vi "commander9.vi"() -> ()   [LabVIEW 2015]
uses:
  <vilib>/National Instruments/NI Dynamixel API/Dynamixel Pro Driver/Controls/Write Select Pro.ctl
  <vilib>/National Instruments/NI Dynamixel API/Dynamixel Pro Driver/Controls/Baudrate Selector.ctl
  G_ALL.vi
  G_LCM.vi
  G_SEN.vi
  <vilib>/National Instruments/NI Dynamixel API/Dynamixel Pro Driver/Write/Write Dynamixel Pro.vi
  <vilib>/National Instruments/NI Dynamixel API/Dynamixel Pro Driver/Helper VIs/Torque Disable.vi
  <vilib>/National Instruments/NI Dynamixel API/Dynamixel Pro Driver/Helper VIs/Torque Enable.vi
  <vilib>/National Instruments/NI Dynamixel API/Dynamixel Pro Driver/Dynamixel Pro Driver.lvlib
panel:
  in  "Mission":i32
  out "size(s)":i32
  in  "shiift torque gain":i32
  out "robotis":refnum<visa-resource-name>
  in  "y 2":dbl=1.0
  in  "y":dbl=0.5 format="%#_13g"
  out "CIPV_dist":dbl
  out "CIPV_SPEED":dbl
  in  "dist_error_gain":dbl=0.5 format="%#_13g"
  in  "Globla y shift":dbl min=-5.0 max=5.0 step=0.1
  in  "d":dbl=-3.5 format="%#_13g"
  in  "car detection":bool
  in  "Velodyne":T1(ring)=enum."Velodyne 64"
  in  "reset path":bool
  in  "shifthold":dbl=0.003
  out "String":string
  out "EURECAR_VISION":T2
  out "count":i32=100
  out "P2V Sign":picture[](array[picture])=[bytes[7530], bytes[7530], bytes[7530], bytes[7530]]
  out "Array 2":picture[](array[picture])
  out "sign 2":picture[](array[picture])=[bytes[7530], bytes[7530], bytes[7530], bytes[7530], bytes[7530], bytes[7530]]
  out "sign":picture[](array[picture])=[bytes[14730], bytes[14730], bytes[14730], bytes[14730], bytes[14730], bytes[14730], bytes[14730]]
  in  "TTL":bool=TRUE
  out "obs shift":dbl format="%.2f"
  in  "lane keep":bool=TRUE
  in  "replay":bool
  in  "Global x shift":dbl min=-5.0 max=5.0 step=1.0
  out "display":u32=33
  out "control":u32=10
  out "lane update":bool=TRUE
  in  "save lcm":bool
  out "LCM Recv Data":string="LCM_SELF_TEST\t2\rIBEO_2202_T\t29020\rSDT_GPS_DATA\t5359\rGGA_1\t5359\rRMC_1\t5359\rMobileye560\t14820\rPOS_T\t116849\rPATH_T\t116934\rCON_T\t116934\rVELO_384\t1693774\rCAN_T\t116936\rSantafe\t116936\r"
  out "GPS DATA 2":T3={"type"="WAAS", "x_lcc"=254.06227375244842, "y_lcc"=-1012.895186102979, "latdev"=0.63, "londev"=0.63, "sats"=12, "gps_l1_ranges"=0, "gps_l1_mask_ranges"=0, "gps_l2_mask_ranges"=0, "Heading"=246.4954324105635, "lon"=127.36372, "lat"=36.36631, "time"="22:33:04.0", "hgps"=245.36, "lag"=0.0, "MAP"="KAIST"} {"lag" format="%#_5g"; "hgps" format="%#_5g"; "lat" format="%#_11g"; "lon" format="%#_11g"; "Heading" format="%#_5g"; "latdev" format="%#_4g"; "londev" format="%#_4g"}
  in  "Obs":bool=TRUE
  in  "Log":bool=TRUE
  out "path":u32=10
  out "sensor":u32=10 format="%02.0f"
  out "Speed limit":dbl=25.0
  out "collision":bool
  in  "Load Path":bool
  in  "Max. Vel.":dbl=10.0 min=-5.0 max=120.0 step=5.0
  out "col":i16(graph)
  out "stop":bool=TRUE
  in  "Reverse":bool
  in  "STOP":bool
  out "Waveform Chart 4":cluster{"auto":i16, "run":i16}(graph)={"auto"=1, "run"=0}
  out "Waveform Chart 3":cluster{"Steer_input":dbl, dbl, "handle":dbl}(graph)={"Steer_input"=-0.0, 31.6, "handle"=6.530305819273729}
  out "Waveform Chart 2":T4(graph)={"VS_des"=0.0, "VS_can"=22.140625, "VS_des"=0.0}
  out "Heading":cluster{"Heading":dbl, "hgps":dbl}(graph)={"Heading"=246.4954324105635, "hgps"=245.36}
  out "XY Graph 2":cluster{"Y":dbl[], "Y":dbl[]}[](graph)=[{"Y"=[254.2844178548139], "Y"=[-1012.8240977739181]}, {"Y"=array[3210 elements], "Y"=array[3210 elements]}, {"Y"=array[3210 elements], "Y"=array[3210 elements]}]
  out "Gauge":cluster{dbl, dbl, dbl}(knob)={0.0, 22.140625, 0.0} scale=-20.0..140.0
  out "Meter":cluster{dbl, dbl, dbl}(knob)={-0.0, 31.6, 6.530305819273729} scale=-550.0..550.0
  out "XY Graph":cluster{"Y":dbl[], "Y":dbl[]}[](graph)=[{"Y"=array[3210 elements], "Y"=array[3210 elements]}, {"Y"=[-0.0, 0.001154394197769193, 0.004617650635850623, 0.010389990872226917, 0.018471784248973222, 0.02886354801042046, 0.041565947468740205, 0.056579796217107514, 0.0739060563904701, 0.0935458389742223, 0.11550040416098284, 0.13977116175580306, 0.16635967162997645, 0.19526764422393228, 0.2264969410994837, 0.26004957554195585, 0.2959277132125635, 0.3341336728515216, 0.374669927032528, 0.417539102969144, 0.4627439833735707, 0.5102875073687159, 0.560172771454063, 0.6124030305261954, 0.6669816989546717, 0.7239123517142048, 0.7831987255740245, 0.8448447203451934, 0.9088544001870815, 0.975231994973953, 1.0439819017227023, 1.1151086860829622, 1.1886170838907617, 1.2645120027869723, 1.342798523901962, 1.42348190360768, 1.5065675753387922, 1.592061151484188, 1.6799684253507792, 1.770295373200753, 1.8630481563645134, 1.9582331234307588, 2.0558568125157564, 2.1559259536137603, 2.258447471030621], "Y"=[0.0, 0.5, 1.0, 1.5, 2.0, 2.5, 3.0, 3.5, 4.0, 4.5, 5.0, 5.5, 6.0, 6.5, 7.0, 7.5, 8.0, 8.5, 9.0, 9.5, 10.0, 10.5, 11.0, 11.5, 12.0, 12.5, 13.0, 13.5, 14.0, 14.5, 15.0, 15.5, 16.0, 16.5, 17.0, 17.5, 18.0, 18.5, 19.0, 19.5, 20.0, 20.5, 21.0, 21.5, 22.0]}, {"Y"=[0.362252581831572], "Y"=[-0.8199241909738847]}, {"Y"=array[210 elements], "Y"=array[210 elements]}, {"Y"=[-0.925, -0.925, -0.925, -0.6775, -0.6775, -0.925, -0.925, -0.925, -0.925, -0.6775, -0.6775, -0.925, -0.925, -0.925, 0.9025, 0.9025, 0.9025, 0.6775, 0.6775, 0.9025, 0.9025, 0.9025, 0.9025, 0.6775, 0.6775, 0.9025, 0.9025, 0.9025, -0.925], "Y"=[-0.75, -0.224, 0.224, 0.224, -0.224, -0.224, 0.224, 2.415, 2.885, 2.885, 2.415, 2.415, 2.885, 3.5, 3.5, 2.885, 2.415, 2.415, 2.885, 2.885, 2.415, 0.224, -0.224, -0.224, 0.224, 0.224, -0.224, -0.75, -0.75]}, {"Y"=[0.171875, 0.15377271904051304, 0.1346290179491043, 0.11445423440635205, 0.09325870609283447, 0.07105277068912982, 0.04784676587581635, 0.02365102933347224, -0.0015241012573242174, -0.02766828821599482, -0.05477119386196136, -0.08282248051464558, -0.11181181049346922, -0.14172884611785413, -0.17256324970722198, -0.20430468358099463, -0.23694281005859374, -0.27046729145944115, -0.30486779010295867, -0.340133968308568, -0.3762554883956909, -0.41322201268374914, -0.4510232034921646, -0.4896487231403589], "Y"=[0.0, 0.5, 1.0, 1.5, 2.0, 2.5, 3.0, 3.5, 4.0, 4.5, 5.0, 5.5, 6.0, 6.5, 7.0, 7.5, 8.0, 8.5, 9.0, 9.5, 10.0, 10.5, 11.0, 11.5]}, {"Y"=[1.796875, 1.778772719040513, 1.7596290179491043, 1.739454234406352, 1.7182587060928345, 1.6960527706891297, 1.6728467658758164, 1.6486510293334722, 1.6234758987426758, 1.5973317117840051, 1.5702288061380387, 1.5421775194853544, 1.513188189506531, 1.483271153882146, 1.452436750292778, 1.4206953164190055, 1.3880571899414063, 1.354532708540559, 1.3201322098970414, 1.284866031691432, 1.248744511604309, 1.2117779873162509, 1.1739767965078354, 1.135351276859641, 1.0959117660522462, 1.0556686017662287, 1.014632121682167, 0.9728126634806396, 0.9302205648422242, 0.8868661634474992], "Y"=[0.0, 0.5, 1.0, 1.5, 2.0, 2.5, 3.0, 3.5, 4.0, 4.5, 5.0, 5.5, 6.0, 6.5, 7.0, 7.5, 8.0, 8.5, 9.0, 9.5, 10.0, 10.5, 11.0, 11.5, 12.0, 12.5, 13.0, 13.5, 14.0, 14.5]}, {"Y"=[-1.453125, -1.471227280959487, -1.4903709820508957, -1.510545765593648, -1.5317412939071655, -1.5539472293108703, -1.5771532341241836, -1.6013489706665278, -1.6265241012573242, -1.6526682882159949, -1.6797711938619613, -1.7078224805146456, -1.736811810493469, -1.766728846117854, -1.797563249707222, -1.8293046835809945, -1.8619428100585937, -1.895467291459441, -1.9298677901029586], "Y"=[0.0, 0.5, 1.0, 1.5, 2.0, 2.5, 3.0, 3.5, 4.0, 4.5, 5.0, 5.5, 6.0, 6.5, 7.0, 7.5, 8.0, 8.5, 9.0]}, {"Y"=[0.171875, 0.2568230007600336, 0.3384052130063493, 0.44574342526006827, 0.5205081969556753, 0.5917680690742042, 0.659409530134929, 0.7229937549325056, 0.7835496148685115, 0.8405449546633443, 0.9258576868463875], "Y"=[-20.239964538708662, -19.725637940364884, -19.211158961966362, -18.6998967366845, -18.19022720070031, -17.681887266143153, -17.17615515566314, -16.67683575591291, -16.176265245349786, -15.679082775270938, -15.183754484614711]}, {"Y"=[7.134647485270904], "Y"=[38.71960961082238]}, {"Y"=array[980 elements], "Y"=array[980 elements]}, {"Y"=[], "Y"=[]}]
  in  "Make WPT":bool
  in  "mission auto":bool
  # "V2I Traffic Signal"
  # "CNN\nSign\nDetection"
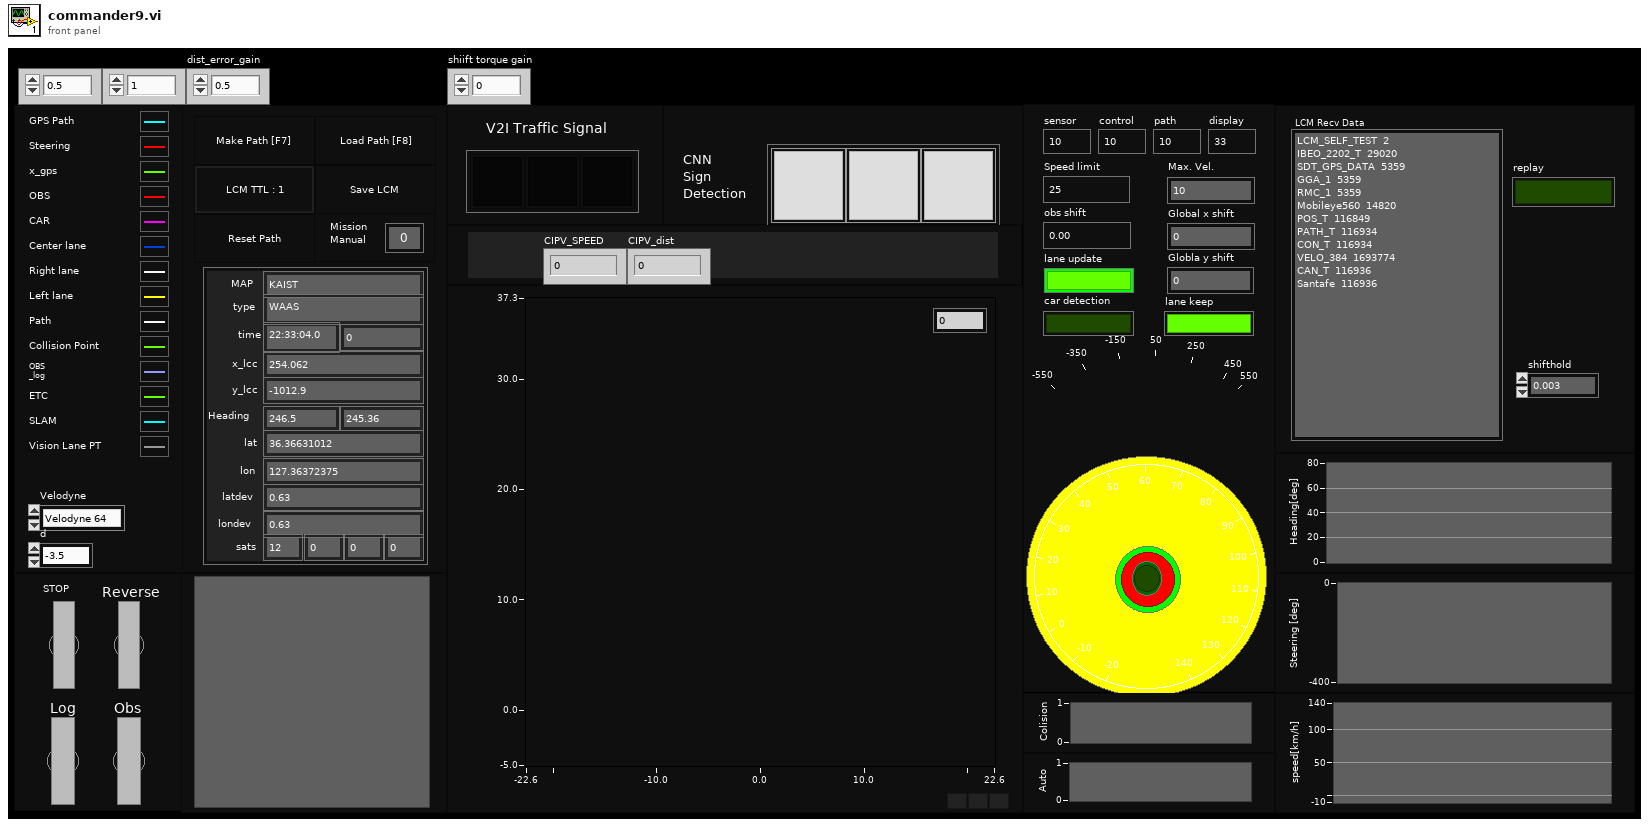
[diagram p1: front panel]
types:
  T1 = enum16{"Velodyne 16", "Velodyne 32", "Velodyne 64"}
  T2 = cluster{"hash":i64, "sys time":i64, "status":i32, "TS_num":i32, "TS_type":i32[], "TS_loc_x":dbl[], "TS_loc_y":dbl[]}
  T3 = cluster{"type":string, "x_lcc":dbl, "y_lcc":dbl, "latdev":sgl, "londev":sgl, "sats":u8, "gps_l1_ranges":u8, "gps_l1_mask_ranges":u8, "gps_l2_mask_ranges":u8, "Heading":dbl, "lon":sgl, "lat":sgl, "time":string, "hgps":dbl, "lag":dbl, "MAP":string}
  T4 = cluster{"VS_des":dbl, "VS_can":dbl, "VS_des":dbl}
  T5 = enum8{"Enabled", "Disabled", "Disabled and Grayed Out"}
  T6 = typedef "Dynamixel Pro Driver.lvlib/Write Select Pro.ctl" = enum16{"ID", "Baud Rate", "Return Delay Time", "Operating mode", "Homing offset", "Moving threshold", "Temperature limit", "Max Voltage Limit", "Min Voltage Limit", "acceleration Limit", "Torque Limit", "Velocity Limit", "Max Position Limit", "Min Position Limit", "External Port Mode 1", "External Port Mode 2", "External Port Mode 3", "External Port Mode 4", "Shutdown", "Torque Enable", "LED RED", "LED GREEN", "LED BLUE", "Velocity I Gain", "Velocity P Gain", "Position P Gain", "Goal Position", "Goal Velocity", "Goal Torque", "Goal Acceleration", "External Port Data 1", "External Port Data 2", "External Port Data 3", "External Port Data 4", "Status Return Level"}
  T7 = typedef "Dynamixel Pro Driver.lvlib/Baudrate Selector.ctl" = enum16{"2400", "57600", "115200", "1000000", "2000000", "3000000", "4000000", "4500000", "10500000"}
  T8 = cluster{"Steer_input":dbl, "Steer_output":dbl, "VS_des":dbl, "VS_can":dbl, "heading":dbl, "auto":bool, "run":bool, "x":dbl, "y":dbl}
  T9 = cluster{"identifier":u32, "timestamp":timestamp, "payload":u8[]}
  T10 = cluster{"hash":i64, "sys time":i64, "size":i32, "data":u8[]}
  T11 = typedef "imagedata.ctl" = cluster{"image type":i32, "image depth":i32, "image":u8[], "mask":u8[], "colors":u32[], "Rectangle":cluster{"left":i16, "top":i16, "right":i16, "bottom":i16}}
  T12 = cluster{"hash":i64, "sys time":i64, "s_lat":dbl, "s_lon":dbl, "d_lat":dbl, "d_lon":dbl, "Message":i64}
  T13 = cluster{"beep":bool, "duration (msec)":u32, "frequency (Hz)":u32}
  T14 = enum32{"Namyang", "Hyundai", "KAIST", "Ajou", "Munji", "Airforce", "Car", "KATRI", "Samsung", "Coex", "Gwangnaru", "Inje", "sinjin", "NAVER"}
  T15 = cluster{"Minimum":dbl, "Minimum":dbl, "Minimum":dbl, "Minimum":dbl, "Minimum":dbl}
  T16 = cluster{"hash":i64, "sys time":i64, "time":dbl, "x":dbl, "y":dbl, "h":dbl, "numSV":i32, "postype":i32, "lag":i32, "hordev":dbl, "lat":dbl, "lon":dbl, "hgt":dbl, "map_idx":i32}
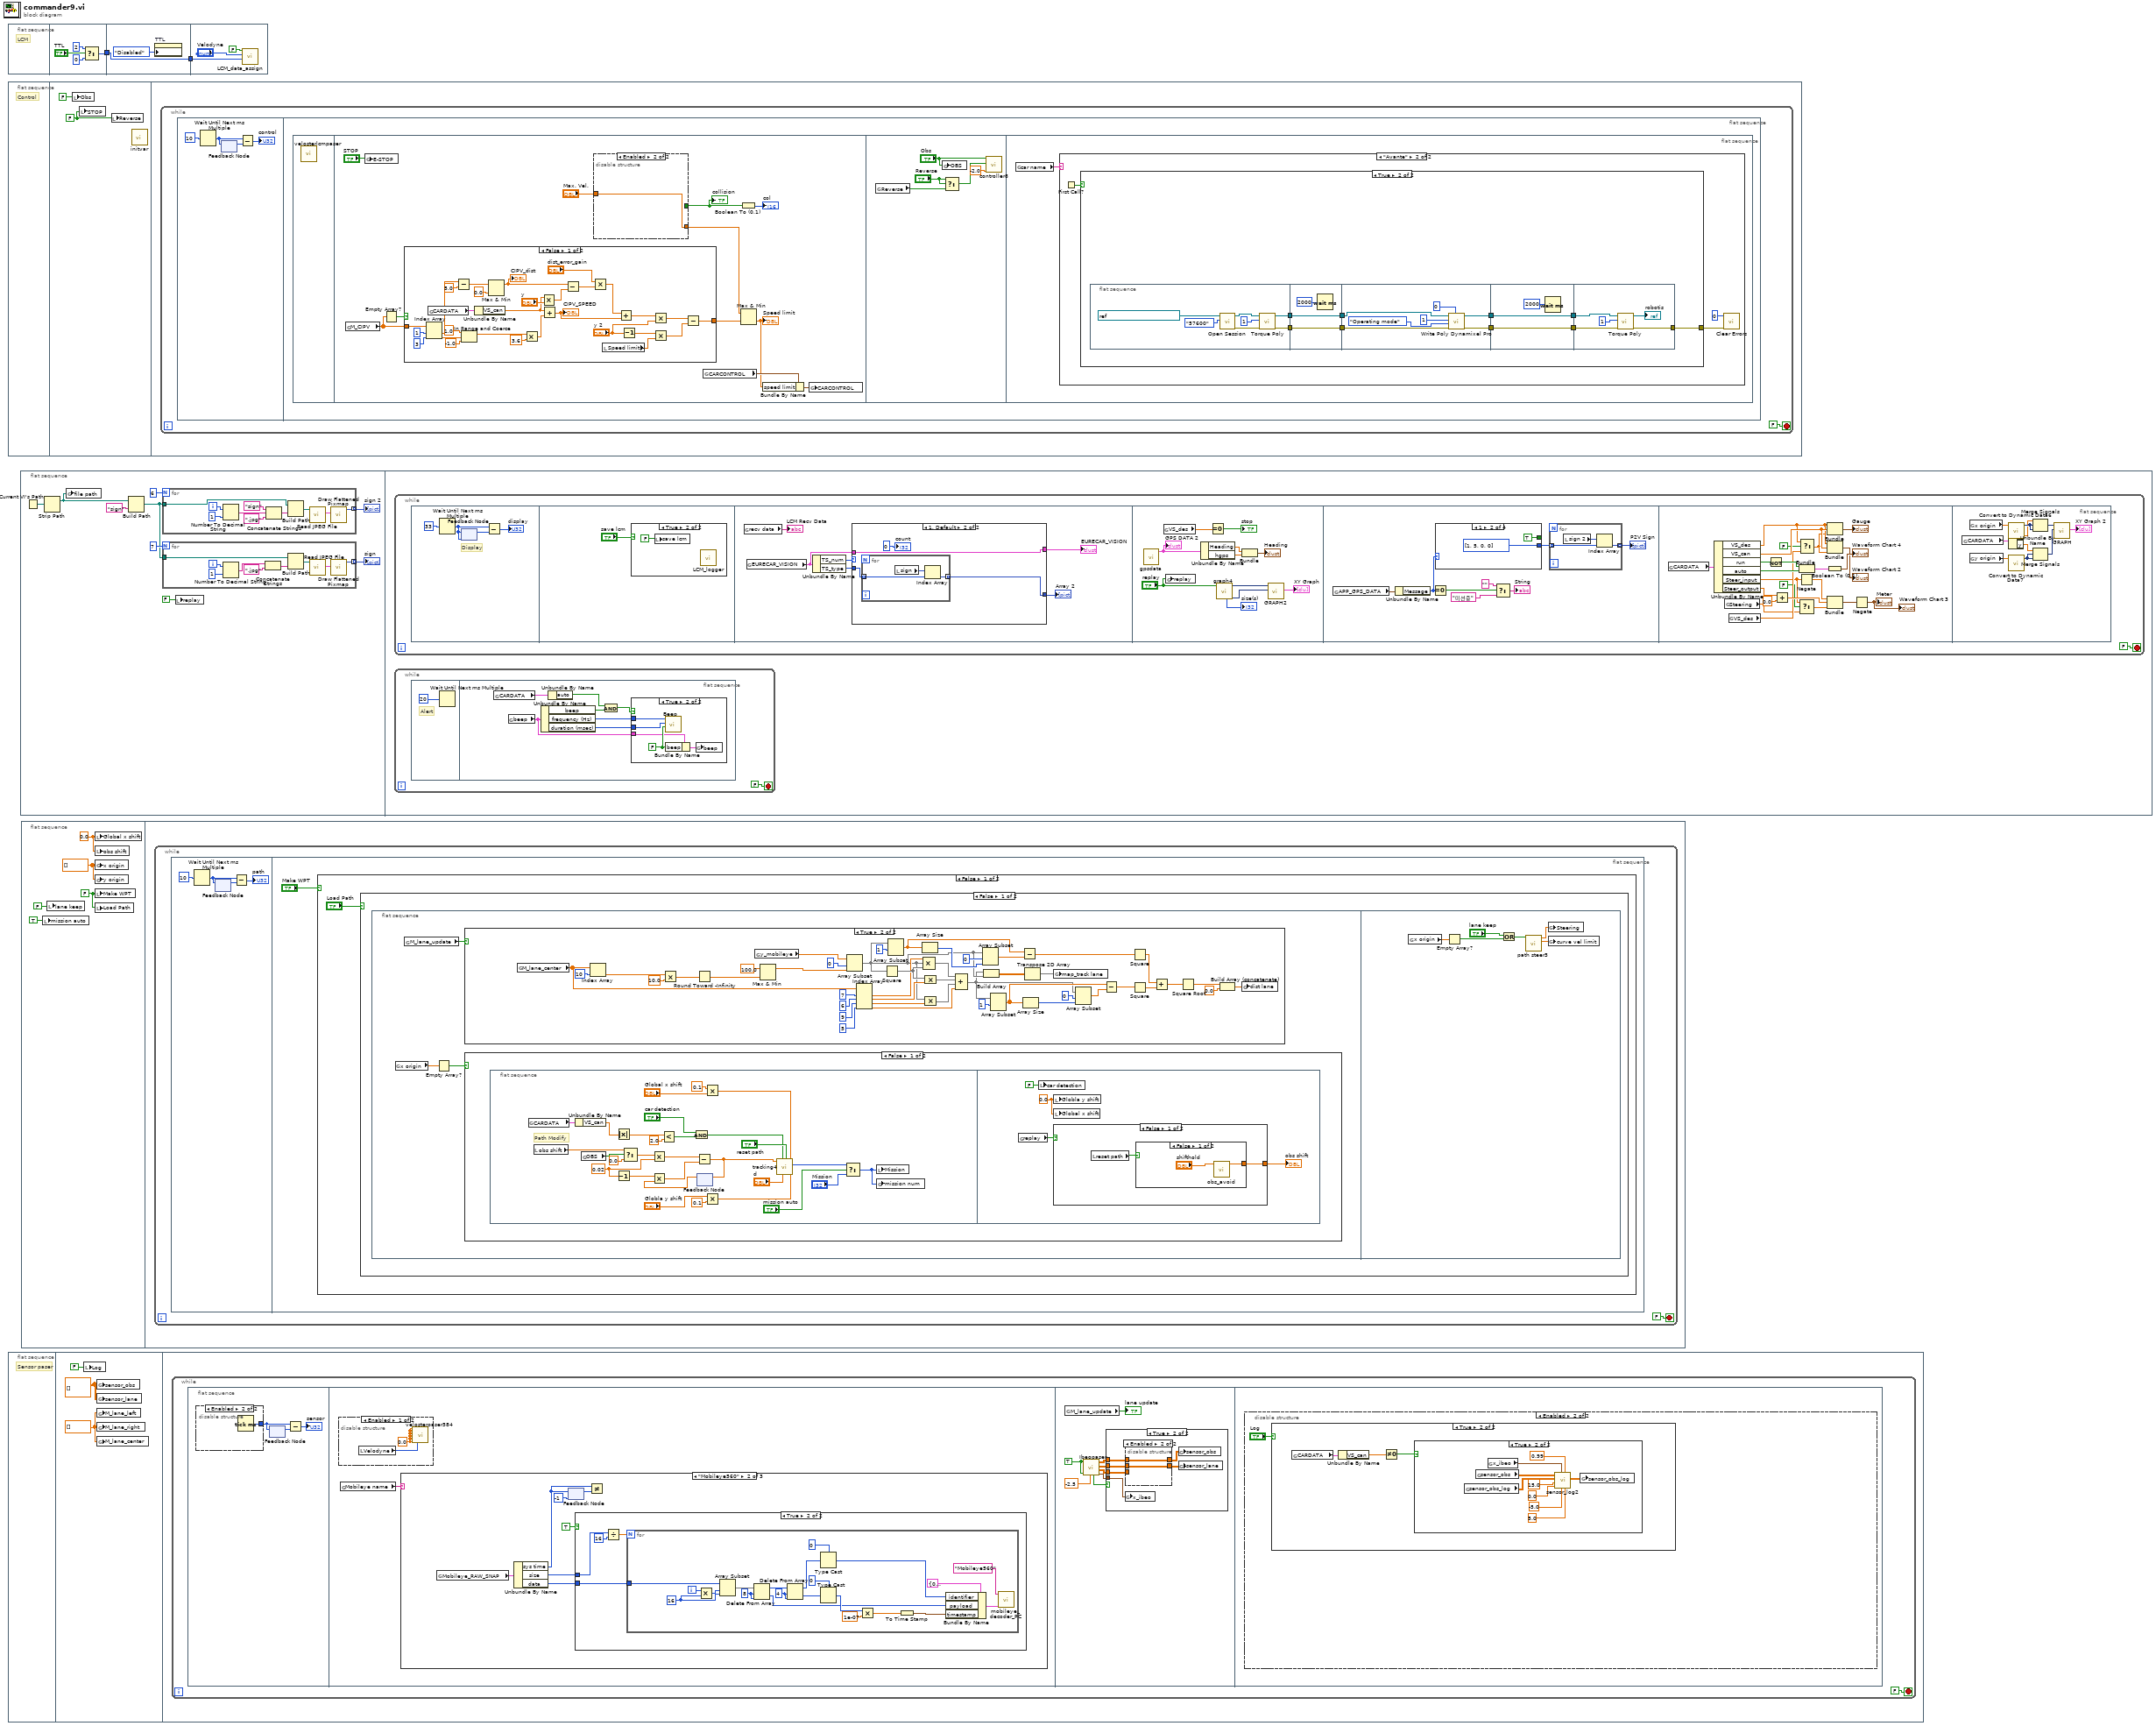
[diagram p0: block diagram]
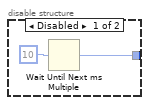
[diagram p2: hidden frame]
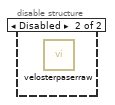
[diagram p3: hidden frame]
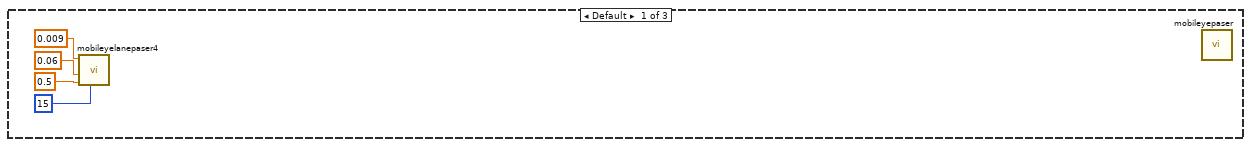
[diagram p4: hidden frame]
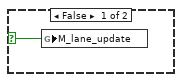
[diagram p5: hidden frame]
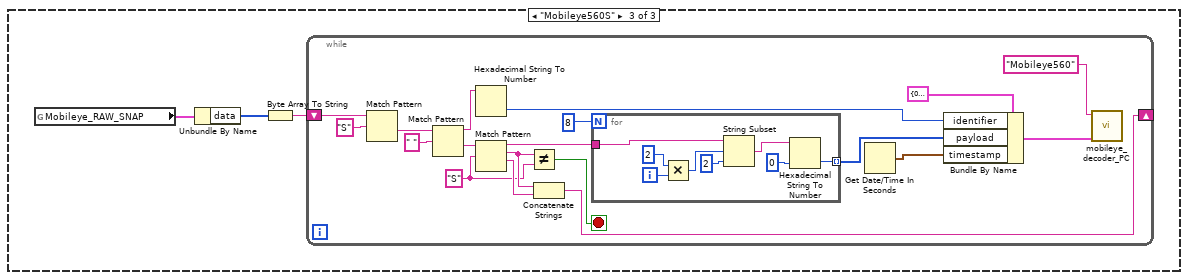
[diagram p6: hidden frame]
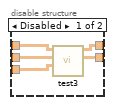
[diagram p8: hidden frame]
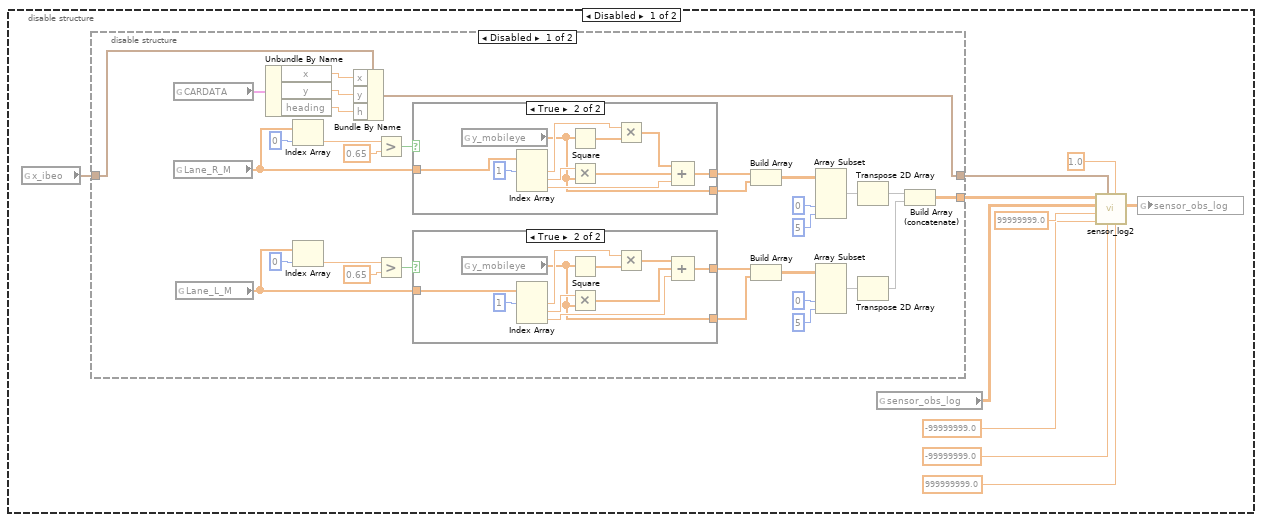
[diagram p9: hidden frame]
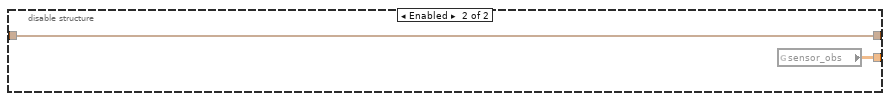
[diagram p12: hidden frame]
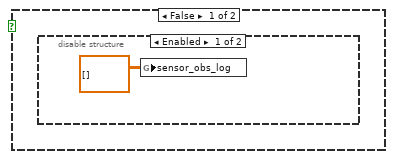
[diagram p13: hidden frame]
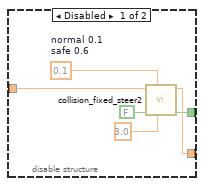
[diagram p16: hidden frame]
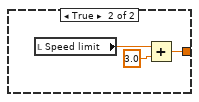
[diagram p17: hidden frame]
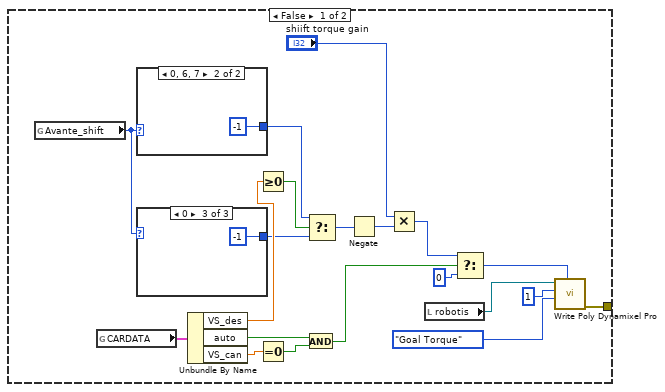
[diagram p19: hidden frame]
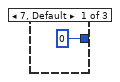
[diagram p20: hidden frame]
diagram:
  n1 = flat-sequence {
    tunnel: [w3] -> w1
    tunnel: [w8] -> w2
    tunnel: w1 -> [w8]
    tunnel: w2 -> [w10]
    frame #0 {
      # "LCM"
    }
    frame #1 {
      n2 = Select(t=u16 2 ("time-to-live"), s="TTL", f=u16 0 ("time-to-live")) -> (s? t:f=w3:u16)
    }
    frame #2 {
      n3 = property on="TTL" class="Bool (strict)"("DisabledEnum"=T5."Disabled" ("Disabled")) -> ()  [unwired: 2 in, 2 out]
    }
    frame #3 {
      n4 = call "LCM_data_assign.vi"("time-to-live"=w10, "Velodyne1"="Velodyne", "velodyne enable"=FALSE) -> ()  [unwired: 9 in]
    }
  }
  n5 = flat-sequence {
    frame #0 {
      # "Control"
    }
    frame #1 {
      w13 = FALSE ("LCM")
      n6 = local write "Obs"(FALSE ("obs")) -> ()
      n7 = local write "STOP"(w13) -> ()
      n8 = local write "Reverse"(w13) -> ()
      n9 = call "initvar.vi"() -> ()  [unwired: 12 in]
    }
    frame #2 {
      n10 = while {
        stop <- FALSE ("Loop 1") stop-if-true
        n11 = flat-sequence {
          frame #0 {
            n12 = Wait Until Next ms Multiple(millisecond multiple=u32 10 ("milliseconds to wait")) -> (millisecond timer value=w15:u32)
            n13 = feedback #1() -> (w16:u32)  [unwired: 1 in]
            n14 = feedback-in #1(w15) -> ()
            n15 = Subtract(x=w15, y=w16) -> (x-y=→"control":u32)
          }
          frame #1 {
            n16 = flat-sequence {
              frame #0 {
                n17 = call "velosterlcmpaser.vi"() -> ()  [unwired: 11 in, 1 out]
              }
              frame #1 {
                n18 = global read "G_SEN.vi" "M_CIPV"() -> (w22:dbl[])
                n19 = global write "G_ALL.vi" "E-STOP"("STOP") -> ()
                n20 = Empty Array?(array=w22) -> (empty?=w23:bool)
                n21 = case shown="False" w23 {
                  tunnel: w22 -> [w65 _]
                  tunnel: [w48 w67] -> w19
                  frame False {
                    n22 = Index Array(array=w65, index #1=1 ("index"), index #2=3 ("index")) -> (element #1=w43:dbl, element #2=w47:dbl)
                    n23 = global read "G_ALL.vi" "CARDATA"() -> (w63:T8)
                    n24 = Subtract(x=w43, y=5.0) -> (x-y=w41:dbl)
                    n25 = In Range and Coerce(upper limit=1.0, x=w47, lower limit=-1.0) -> (coerced(x)=w44:dbl)  [unwired: 1 out]
                    n26 = Unbundle By Name(w63) -> ("VS_can"=w37:dbl)
                    n27 = Max & Min(x=w41, y=0.0) -> (max(x,y)=w39:dbl)  [unwired: 1 out]
                    "CIPV_dist" <- w39
                    n28 = Multiply(x=w44, y=3.6) -> (x*y=w57:dbl)
                    n29 = Multiply(x=w37, y="y") -> (x*y=w55:dbl)
                    n30 = Add(x=w37, y=w57) -> (x+y=w38:dbl)
                    "CIPV_SPEED" <- w38
                    n31 = Subtract(x=w39, y=w55) -> (x-y=w58:dbl)
                    n32 = Multiply(x="dist_error_gain", y=w58) -> (x*y=w60:dbl)
                    n33 = local read "Speed limit"() -> (w51:dbl)
                    n34 = Add(x=w60, y=w38) -> (x+y=w54:dbl)
                    n35 = Decrement(x="y 2") -> (x-1=w52:dbl)
                    n36 = Multiply(x=w54, y="y 2") -> (x*y=w49:dbl)
                    n37 = Multiply(x=w52, y=w51) -> (x*y=w50:dbl)
                    n38 = Subtract(x=w49, y=w50) -> (x-y=w48:dbl)
                  }
                  frame True {
                    n39 = local read "Speed limit"() -> (w68:dbl)
                    n40 = Add(x=w68, y=3.0) -> (x+y=w67:dbl)
                  }
                }
                n41 = disable-structure shown="Enabled" {
                  disable-tunnel: "Max. Vel." -> [w35 w36]
                  disable-tunnel: [w31 _] -> w27
                  disable-tunnel: [w30 w36] -> w21
                  frame Disabled {
                    w32 = 0.1  # normal 0.1 safe 0.6
                    n42 = call "collision_fixed_steer2.vi"("safe  dist"=3.0, "y"=w32, "obsclose"=FALSE, "Max. Vel."=w35) -> ("collision"=w31:bool, "speed limit"=w30:dbl)  [unwired: 5 in, 1 out]
                  }
                  frame Enabled {
                  }
                }
                "collision" <- w27
                n43 = global read "G_ALL.vi" "CARCONTROL"() -> (w25:cluster{"speed path":dbl, "speed limit":dbl})
                n44 = Boolean To (0,1)(Boolean=w27) -> (0, 1=→"col":i16)
                n45 = Max & Min(x=w21, y=w19) -> (min(x,y)=w20:dbl)  [unwired: 1 out]
                "Speed limit" <- w20
                n46 = Bundle By Name(cluster=w25, "speed limit"=w20) -> (w24:cluster{"speed path":dbl, "speed limit":dbl})
                n47 = global write "G_ALL.vi" "CARCONTROL"(w24) -> ()
              }
              frame #2 {
                n48 = global read "G_ALL.vi" "Reverse"() -> (w70:bool)
                n49 = global write "G_ALL.vi" "OBS"("Obs") -> ()
                n50 = Select(t="Reverse", s="Reverse", f=w70) -> (s? t:f=w72:bool)
                n51 = call "controller8.vi"("Neg max speed"=-2.0, "reverse"=w72, "obs"="Obs") -> ()  [unwired: 9 in]
              }
              frame #3 {
                n52 = global read "G_LCM.vi" "car name"() -> (w74:string)
                n53 = case shown="\"Avante\"" w74 {
                  frame Default {
                  }
                  frame "Avante" {
                    n54 = First Call?() -> (First Call?: T/F=w77:bool)
                    n55 = case shown="True" w77 {
                      tunnel: [w97 w103] -> w76
                      frame False {
                        n56 = global read "G_ALL.vi" "Avante_shift"() -> (w85:u8)
                        n57 = global read "G_ALL.vi" "CARDATA"() -> (w90:T8)
                        n58 = case shown="0, 6, 7" w85 {
                          tunnel: [0 -1] -> w83
                          frame 5, Default {
                          }
                          frame 0, 6, 7 {
                          }
                        }
                        n59 = case shown="0" w85 {
                          tunnel: [0 1 -1] -> w82
                          frame 7, Default {
                          }
                          frame 5, 6 {
                          }
                          frame 0 {
                          }
                        }
                        n60 = Unbundle By Name(w90) -> ("VS_des"=w86:dbl, "auto"=w88:bool, "VS_can"=w89:dbl)
                        n61 = Greater Or Equal To 0?(x=w86) -> (x >= 0?=w84:bool)
                        n62 = Equal To 0?(x=w89) -> (x = 0?=w87:bool)
                        n63 = And(x=w88, y=w87) -> (x .and. y?=w96:bool)
                        n64 = Select(t=w83, s=w84, f=w82) -> (s? t:f=w81:i32)
                        n65 = Negate(x=w81) -> (-x=w80:i32)
                        n66 = Multiply(x="shiift torque gain", y=w80) -> (x*y=w92:i32)
                        n67 = local read "robotis"() -> (w79:refnum<visa-resource-name>)
                        n68 = Select(t=w92, s=w96, f=0) -> (s? t:f=w93:i32)
                        n69 = call-poly <vilib>:"Write Poly Dynamixel Pro.vi"("Value"=w93, "Operation"=Write_Select_Pro."Goal Torque", "ID"=u8 1, "VISA Refnum in"=w79) -> ("error out"=w97:errorcluster)  [unwired: 6 in, 1 out]
                      }
                      frame True {
                        n70 = flat-sequence {
                          tunnel: [w114] -> w111
                          tunnel: [w113] -> w110
                          tunnel: [w121] -> w109
                          tunnel: w111 -> [w121]
                          tunnel: [w120] -> w108
                          tunnel: w110 -> [w120]
                          tunnel: [w125] -> w107
                          tunnel: w109 -> [w127]
                          tunnel: w108 -> [w126]
                          tunnel: [w124] -> w106
                          tunnel: w107 -> [w131]
                          tunnel: [w131] -> w105
                          tunnel: [w130] -> w104
                          tunnel: w106 -> [w130]
                          tunnel: [w134] -> w103
                          tunnel: w105 -> [w136]
                          tunnel: w104 -> [w135]
                          frame #0 {
                            n71 = call <vilib>:"Open Session.vi"("Baud Rate"=Baudrate_Selector."57600", "VISA resource name"=refnum<visa-resource-name> "COM5") -> ("error out"=w117:errorcluster, "VISA Refnum out"=w118:refnum<visa-resource-name>)  [unwired: 8 in]
                            n72 = call-poly <vilib>:"Torque Poly.vi"("error in (no error)"=w117, "ID"=u8 1, "VISA Refnum in"=w118) -> ("error out"=w113:errorcluster, "VISA Refnum out"=w114:refnum<visa-resource-name>)  [unwired: 7 in]
                          }
                          frame #1 {
                            n73 = Wait (ms)(milliseconds to wait=u32 2000) -> ()  [unwired: 1 out]
                          }
                          frame #2 {
                            n74 = call-poly <vilib>:"Write Poly Dynamixel Pro.vi"("Value"=0, "error in (no error)"=w126, "Operation"=Write_Select_Pro."Operating mode", "ID"=u8 1, "VISA Refnum in"=w127) -> ("error out"=w124:errorcluster, "VISA Refnum out"=w125:refnum<visa-resource-name>)  [unwired: 5 in]
                          }
                          frame #3 {
                            n75 = Wait (ms)(milliseconds to wait=u32 2000) -> ()  [unwired: 1 out]
                          }
                          frame #4 {
                            n76 = call-poly <vilib>:"Torque Poly.vi"("error in (no error)"=w135, "ID"=u8 1, "VISA Refnum in"=w136) -> ("error out"=w134:errorcluster, "VISA Refnum out"=→"robotis":refnum<visa-resource-name>)  [unwired: 7 in]
                          }
                        }
                      }
                    }
                    n77 = call <vilib>:"Clear Errors.vi"("error in (no error)"=w76, "specific error code to clear (0: all)"=0) -> ()  [unwired: 4 in, 2 out]
                  }
                }
              }
            }
          }
        }
      }
    }
  }
  n78 = flat-sequence {
    frame #0 {
      # "Sensor paser"
    }
    frame #1 {
      w137 = dbl[][] [] ("M_lane_left")
      w138 = dbl[] [] ("M_lane_left")
      n79 = local write "Log"(FALSE ("obs")) -> ()
      n80 = global write "G_SEN.vi" "sensor_obs"(w137) -> ()
      n81 = global write "G_SEN.vi" "sensor_lane"(w137) -> ()
      n82 = global write "G_SEN.vi" "M_lane_left"(w138) -> ()
      n83 = global write "G_SEN.vi" "M_lane_right"(w138) -> ()
      n84 = global write "G_SEN.vi" "M_lane_center"(w138) -> ()
    }
    frame #2 {
      n85 = while {
        stop <- FALSE ("Loop 4") stop-if-true
        n86 = flat-sequence {
          frame #0 {
            n87 = disable-structure shown="Enabled" {
              disable-tunnel: [w144 w146] -> w141
              frame Disabled {
                n88 = Wait Until Next ms Multiple(millisecond multiple=u32 10 ("milliseconds to wait")) -> (millisecond timer value=w144:u32)
              }
              frame Enabled {
                n89 = Tick Count (ms)() -> (millisecond timer value=w146:u32)
              }
            }
            n90 = feedback #2() -> (w143:u32)  [unwired: 1 in]
            n91 = feedback-in #2(w141) -> ()
            n92 = Subtract(x=w141, y=w143) -> (x-y=→"sensor":u32)
          }
          frame #1 {
            n93 = disable-structure shown="Enabled" {
              frame Enabled {
                w148 = 0.0 ("roll")
                n94 = local read "Velodyne"() -> (w149:T1)
                n95 = call "velosterpaser384.vi"("roll"=w148, "pitch"=w148, "heading"=w148, "dX"=w148, "dY"=w148, "dZ"=w148, "Velodyne"=w149) -> ()  [unwired: 12 in, 1 out]
              }
              frame Disabled {
                n96 = call "velosterpaserraw.vi"() -> ()  [unwired: 20 in]
              }
            }
            n97 = global read "G_LCM.vi" "Mobileye name"() -> (w147:string)
            n98 = case shown="\"Mobileye560\"" w147 {
              frame Default {
                n99 = call "mobileyelanepaser4.vi"("count hold"=u64 15, "thresh  c"=0.5, "thresh  b"=0.06 ("thresh 2"), "thresh r"=0.009 ("y")) -> ()  [unwired: 4 in, 4 out]
                n100 = call "mobileyepaser.vi"() -> ()  [unwired: 11 in, 1 out]
              }
              frame "Mobileye560" {
                n101 = global read "G_LCM.vi" "Mobileye_RAW_SNAP"() -> (w158:T10)
                n102 = Unbundle By Name(w158) -> ("sys time"=w156:i64, "size"=w159:i32, "data"=w160:u8[])
                n103 = feedback-in #3(w156) -> ()
                n104 = feedback #3(i64 -1 ("sys time")) -> (w155:i64)
                n105 = case shown="True" TRUE {
                  selector: TRUE -> [w161 _]
                  tunnel: w160 -> [_ w165]
                  tunnel: w159 -> [_ w162]
                  frame False {
                    n106 = global write "G_SEN.vi" "M_lane_update"(w161) -> ()
                  }
                  frame True {
                    n107 = Divide(x=w162, y=16) -> (x/y=w164:dbl)
                    n108 = for {
                      N: w164 -> [_]
                      tunnel: w165 -> [w186]
                      i -> [w185]
                      w178 = 4 ("length")
                      w176 = 8 ("index")
                      w184 = 16 ("y")
                      n109 = Multiply(x=w185, y=w184) -> (x*y=w183:i32)
                      n110 = Array Subset(array=w186, index=w183, length=w184) -> (w168:u8[])
                      n111 = Delete From Array(array=w168, length=w176, index=w176) -> (deleted portion=w169:u8[], array with subset deleted=w177:u8[])
                      n112 = Delete From Array(array=w177, length=w178, index=w178) -> (deleted portion=w182:u8[], array with subset deleted=w179:u8[])
                      n113 = Type Cast(type=u32 0, x=w179) -> (*(type *) &x=w170:u32)
                      n114 = Type Cast(type=u32 0, x=w182) -> (*(type *) &x=w171:u32)
                      n115 = Multiply(x=w171, y=1e-07) -> (x*y=w174:dbl)
                      n116 = To Time Stamp(1:w174) -> (0:w173:timestamp)
                      n117 = Bundle By Name(cluster=T9 {"identifier"=0, "timestamp"=timestamp(0 s since 1904-01-01), "payload"=[]} ("can cluster"), "identifier"=w170, "payload"=w169, "timestamp"=w173) -> (w167:T9)
                      n118 = call "mobileye_decoder_PC.vi"("can cluster"=w167, "name"="Mobileye560") -> ()  [unwired: 10 in]
                    }
                  }
                }
                n119 = Not Equal?(x=w156, y=w155) -> ()  [unwired: 1 out]
              }
              frame "Mobileye560S" {
                n120 = global read "G_LCM.vi" "Mobileye_RAW_SNAP"() -> (w189:T10)
                n121 = Unbundle By Name(w189) -> ("data"=w188:u8[])
                n122 = Byte Array To String(unsigned byte array=w188) -> (string=w187:string)
                n123 = while {
                  shift-right: [w192] -> _
                  shift-left: w187 -> [w194]
                  stop <- w193 stop-if-true
                  w198 = "S" ("regular expression")
                  n124 = Match Pattern(string=w194, regular expression="S") -> (after substring=w207:string)  [unwired: 1 in, 3 out]
                  n125 = Match Pattern(string=w207, regular expression=" ") -> (before substring=w205:string, after substring=w203:string)  [unwired: 1 in, 2 out]
                  n126 = Hexadecimal String To Number(string=w205) -> (number=w196:u32)  [unwired: 2 in, 1 out]
                  n127 = Match Pattern(string=w203, regular expression=w198) -> (before substring=w202:string, match substring=w199:string, after substring=w200:string)  [unwired: 1 in, 1 out]
                  n128 = Not Equal?(x=w199, y=w198) -> (x != y?=w193:bool)
                  n129 = Concatenate Strings(w199, w200) -> (w192:string)
                  n130 = for {
                    N: 8 -> [_]
                    tunnel: w202 -> [w216]
                    tunnel: [w212] -> w195 mode=indexing
                    i -> [w211]
                    n131 = Multiply(x=2, y=w211) -> (x*y=w214:i32)
                    n132 = String Subset(string=w216, offset (0)=w214, length (rest)=2 ("length (rest)")) -> (substring=w209:string)
                    n133 = Hexadecimal String To Number(string=w209, default (0uL)=u8 0) -> (number=w212:u8)  [unwired: 1 in, 1 out]
                  }
                  n134 = Get Date/Time In Seconds() -> (seconds since 1Jan1904=w201:timestamp)
                  n135 = Bundle By Name(cluster=T9 {"identifier"=0, "timestamp"=timestamp(0 s since 1904-01-01), "payload"=[]} ("can cluster"), "identifier"=w196, "payload"=w195, "timestamp"=w201) -> (w190:T9)
                  n136 = call "mobileye_decoder_PC.vi"("can cluster"=w190, "name"="Mobileye560") -> ()  [unwired: 10 in]
                }
              }
            }
          }
          frame #2 {
            w219 = TRUE ("Sensor [F12]")
            n137 = global read "G_SEN.vi" "M_lane_update"() -> (→"lane update":bool)
            n138 = call "Ibeopaser.vi"("theta"=-2.5, "Hide Transparent"=w219, "Sensor [F12]"=w219) -> ("x_sensor"=w223:cluster{"idx":i32, "x":dbl, "y":dbl, "h":dbl}, "etc"=w221:dbl[][], "lane"=w222:dbl[][], "obs"=w224:dbl[][], "update"=w220:bool)  [unwired: 4 in]
            n139 = case shown="True" w220 {
              tunnel: w224 -> [_ w230]
              tunnel: w223 -> [_ w225]
              tunnel: w222 -> [_ w227]
              tunnel: w221 -> [_ w228]
              frame False {
              }
              frame True {
                n140 = disable-structure shown="Enabled" {
                  disable-tunnel: w230 -> [w235 w237]
                  disable-tunnel: [w234 w237] -> w229
                  disable-tunnel: w228 -> [w233 _]
                  disable-tunnel: w227 -> [w232 w236]
                  disable-tunnel: [w231 w236] -> w226
                  frame Disabled {
                    n141 = call "test3.vi"("sensor_all"=w233, "sensor_lane"=w232, "sensor_obs"=w235) -> ("lane"=w231:dbl[][], "obs"=w234:dbl[][])  [unwired: 6 in, 1 out]
                  }
                  frame Enabled {
                  }
                }
                n142 = global write "G_ALL.vi" "x_ibeo"(w225) -> ()
                n143 = global write "G_SEN.vi" "sensor_obs"(w229) -> ()
                n144 = global write "G_SEN.vi" "sensor_lane"(w226) -> ()
              }
            }
          }
          frame #3 {
            n145 = disable-structure shown="Enabled" {
              frame Disabled {
                n146 = global read "G_ALL.vi" "x_ibeo"() -> (w239:cluster{"idx":i32, "x":dbl, "y":dbl, "h":dbl})
                n147 = disable-structure shown="Disabled" {
                  disable-tunnel: [w266 w300] -> w240
                  disable-tunnel: w239 -> [w252 w299]
                  disable-tunnel: [w251 w299] -> w238
                  frame Disabled {
                    n148 = global read "G_ALL.vi" "CARDATA"() -> (w253:T8)
                    n149 = global read "G_SEN.vi" "Lane_R_M"() -> (w275:dbl[])
                    n150 = global read "G_SEN.vi" "Lane_L_M"() -> (w272:dbl[])
                    n151 = Unbundle By Name(w253) -> ("x"=w250:dbl, "y"=w249:dbl, "heading"=w248:dbl)
                    n152 = Index Array(array=w275, index=0) -> (element=w277:dbl)
                    n153 = Index Array(array=w272, index=0) -> (element=w270:dbl)
                    n154 = Bundle By Name(cluster=w252, "x"=w250, "y"=w249, "h"=w248) -> (w251:cluster{"idx":i32, "x":dbl, "y":dbl, "h":dbl})
                    n155 = Greater?(x=w277, y=0.65) -> (0:w276:bool)
                    n156 = Greater?(x=w270, y=0.65) -> (0:w271:bool)
                    n157 = case shown="True" w276 {
                      tunnel: w275 -> [_ w290]
                      tunnel: [_ w291] -> w261
                      tunnel: [_ w289] -> w260
                      frame False {
                      }
                      frame True {
                        n158 = global read "G_SEN.vi" "y_mobileye"() -> (w289:dbl[])
                        n159 = Index Array(array=w290, index #1=1 ("index")) -> (element #1=w296:dbl, element #2=w295:dbl, element #3=w292:dbl)  [unwired: 2 in]
                        n160 = Square(x=w289) -> (x^2=w297:dbl[])
                        n161 = Multiply(x=w295, y=w289) -> (x*y=w293:dbl[])
                        n162 = Multiply(x=w296, y=w297) -> (x*y=w294:dbl[])
                        n163 = Compound Arithmetic op=ADD(w294, w293, w292) -> (w291:dbl[])
                      }
                    }
                    n164 = case shown="True" w271 {
                      tunnel: w272 -> [_ w280]
                      tunnel: [_ w281] -> w259
                      tunnel: [_ w279] -> w258
                      frame False {
                      }
                      frame True {
                        n165 = global read "G_SEN.vi" "y_mobileye"() -> (w279:dbl[])
                        n166 = Index Array(array=w280, index #1=1 ("index")) -> (element #1=w286:dbl, element #2=w285:dbl, element #3=w282:dbl)  [unwired: 2 in]
                        n167 = Square(x=w279) -> (x^2=w287:dbl[])
                        n168 = Multiply(x=w285, y=w279) -> (x*y=w283:dbl[])
                        n169 = Multiply(x=w286, y=w287) -> (x*y=w284:dbl[])
                        n170 = Compound Arithmetic op=ADD(w284, w283, w282) -> (w281:dbl[])
                      }
                    }
                    n171 = Build Array(w261, w260) -> (w265:dbl[][])
                    n172 = Build Array(w259, w258) -> (w263:dbl[][])
                    n173 = Array Subset(array=w265, index (col)=0 ("index"), length (col)=5 ("length")) -> (w264:dbl[][])  [unwired: 2 in]
                    n174 = Array Subset(array=w263, index (col)=0 ("index"), length (col)=5 ("length")) -> (w262:dbl[][])  [unwired: 2 in]
                    n175 = Transpose 2D Array(2D array=w264) -> (transposed array=w268:dbl[][])
                    n176 = Transpose 2D Array(2D array=w262) -> (transposed array=w267:dbl[][])
                    n177 = Build Array (concatenate)(w268, w267) -> (w266:dbl[][])
                  }
                  frame Enabled {
                    n178 = global read "G_SEN.vi" "sensor_obs"() -> (w300:dbl[][])
                  }
                }
                n179 = global read "G_SEN.vi" "sensor_obs_log"() -> (w244:dbl[][])
                n180 = call "sensor_log2.vi"("xmax"=999999999.0, "FF"=1.0 ("t"), "xmin"=-99999999.0, "x_sensor"=w238, "ymin"=-99999999.0, "ymax"=99999999.0, "sensor_log in"=w244, "sensor_obs"=w240) -> ("sensor_log out"=w243:dbl[][])  [unwired: 3 in]
                n181 = global write "G_SEN.vi" "sensor_obs_log"(w243) -> ()
              }
              frame Enabled {
                n182 = case shown="True" "Log" {
                  frame False {
                    n183 = disable-structure shown="Enabled" {
                      frame Enabled {
                        n184 = global write "G_SEN.vi" "sensor_obs_log"(dbl[][] [] ("sensor_obs_log")) -> ()
                      }
                      frame Disabled {
                      }
                    }
                  }
                  frame True {
                    n185 = global read "G_ALL.vi" "CARDATA"() -> (w303:T8)
                    n186 = Unbundle By Name(w303) -> ("VS_can"=w305:dbl)
                    n187 = Not Equal To 0?(x=w305) -> (x != 0?=w304:bool)
                    n188 = case shown="True" w304 {
                      frame False {
                      }
                      frame True {
                        n189 = global read "G_SEN.vi" "sensor_obs_log"() -> (w309:dbl[][])
                        n190 = global read "G_SEN.vi" "sensor_obs"() -> (w310:dbl[][])
                        n191 = global read "G_ALL.vi" "x_ibeo"() -> (w306:cluster{"idx":i32, "x":dbl, "y":dbl, "h":dbl})
                        n192 = call "sensor_log2.vi"("xmax"=5.0, "FF"=0.99 ("t"), "xmin"=-5.0, "x_sensor"=w306, "ymin"=0.0, "ymax"=15.0, "sensor_log in"=w309, "sensor_obs"=w310) -> ("sensor_log out"=w308:dbl[][])  [unwired: 3 in]
                        n193 = global write "G_SEN.vi" "sensor_obs_log"(w308) -> ()
                      }
                    }
                  }
                }
              }
            }
          }
        }
      }
    }
  }
  n194 = flat-sequence {
    frame #0 {
      n195 = Current VI's Path() -> (path=w322:path)
      n196 = Strip Path(path=w322) -> (stripped path=w315:path)  [unwired: 1 out]
      n197 = global write "G_ALL.vi" "file path"(w315) -> ()
      n198 = Build Path(base path=w315, name or relative path="sign") -> (appended path=w316:path)
      n199 = for {
        N: 6 -> [_]
        tunnel: [w332] -> w318 mode=indexing
        tunnel: w316 -> [w327]
        i -> [w331]
        n200 = Number To Decimal String(number=w331, width (-)=i16 1) -> (decimal integer string=w329:string)
        n201 = Concatenate Strings("sign" ("string"), w329, ".jpg") -> (w326:string)
        n202 = Build Path(base path=w327, name or relative path=w326) -> (appended path=w325:path)
        n203 = call <vilib>:"Read JPEG File.vi"("path to JPEG file"=w325) -> ("image data"=w333:T11)  [unwired: 8 in, 2 out]
        n204 = call <vilib>:"Draw Flattened Pixmap.vi"("image data"=w333) -> ("new picture"=w332:picture)  [unwired: 8 in]
      }
      "sign 2" <- w318
      n205 = for {
        N: 7 -> [_]
        tunnel: [w341] -> w319 mode=indexing
        tunnel: w316 -> [w336]
        i -> [w340]
        n206 = Number To Decimal String(number=w340, width (-)=i16 1) -> (decimal integer string=w338:string)
        n207 = Concatenate Strings(w338, ".jpg") -> (w335:string)
        n208 = Build Path(base path=w336, name or relative path=w335) -> (appended path=w334:path)
        n209 = call <vilib>:"Read JPEG File.vi"("path to JPEG file"=w334) -> ("image data"=w342:T11)  [unwired: 8 in, 2 out]
        n210 = call <vilib>:"Draw Flattened Pixmap.vi"("image data"=w342) -> ("new picture"=w341:picture)  [unwired: 8 in]
      }
      "sign" <- w319
      n211 = local write "replay"(FALSE ("replay")) -> ()
    }
    frame #1 {
      n212 = while {
        stop <- FALSE ("Loop 2") stop-if-true
        n213 = flat-sequence {
          frame #0 {
            # "Display"
            n214 = Wait Until Next ms Multiple(millisecond multiple=u32 33 ("milliseconds to wait")) -> (millisecond timer value=w358:u32)
            n215 = feedback #4(w358) -> (w360:u32)
            n216 = feedback-in #4(w358) -> ()
            n217 = Subtract(x=w358, y=w360) -> (x-y=→"display":u32)
          }
          frame #1 {
            n218 = case shown="True" "save lcm" {
              frame False {
              }
              frame True {
                n219 = local write "save lcm"(FALSE ("save lcm")) -> ()
                n220 = call "LCM_logger.vi"() -> ()  [unwired: 12 in]
              }
            }
          }
          frame #2 {
            n221 = global read "G_LCM.vi" "recv data"() -> (→"LCM Recv Data":string)
            n222 = global read "G_LCM.vi" "EURECAR_VISION"() -> (w366:T2)
            n223 = Unbundle By Name(w366) -> ("TS_num"=w369:i32, "TS_type"=w368:i32[])
            n224 = case shown="1, Default" w369 {
              tunnel: w368 -> [_ w384]
              tunnel: [w377 w383] -> w367
              tunnel: w366 -> [_ w381]
              tunnel: [w370 w381] -> w365
              frame 0 {
                w379 = 100 ("x")
                n225 = local read "count"() -> (w380:i32)
                n226 = Increment(x=w380) -> (x+1=w375:i32)
                n227 = Max & Min(x=w379, y=w375) -> (min(x,y)=w374:i32)  [unwired: 1 out]
                n228 = local read "EURECAR_VISION"() -> (w371:T2)
                n229 = local write "count"(w374) -> ()
                n230 = Equal?(x=w379, y=w374) -> (x = y?=w373:bool)
                n231 = local read "Array 2"() -> (w376:picture[])
                n232 = Select(t=T2 {"hash"=0, "sys time"=0, "status"=0, "TS_num"=0, "TS_type"=[], "TS_loc_x"=[], "TS_loc_y"=[]} ("EURECAR_VISION"), s=w373, f=w371) -> (s? t:f=w370:T2)
                n233 = Select(t=picture[] [], s=w373, f=w376) -> (s? t:f=w377:picture[])
              }
              frame 1, Default {
                n234 = for {
                  tunnel: w384 -> [w386] mode=indexing
                  tunnel: [w385] -> w383 mode=indexing
                  n235 = local read "sign"() -> (w387:picture[])
                  n236 = Index Array(array=w387, index=w386) -> (element=w385:picture)
                }
                "count" <- 0 ("Numeric Control")
              }
            }
            "Array 2" <- w367
            "EURECAR_VISION" <- w365
          }
          frame #3 {
            n237 = call "gpsdata.vi"() -> ("GPS DATA 2"=w395:T3)  [unwired: 11 in]
            "GPS DATA 2" <- w395
            n238 = global read "G_ALL.vi" "VS_des"() -> (w389:dbl)
            n239 = global write "G_ALL.vi" "replay"("replay") -> ()
            n240 = Unbundle By Name(w395) -> ("Heading"=w397:dbl, "hgps"=w396:dbl)
            n241 = Equal To 0?(x=w389) -> (x = 0?=→"stop":bool)
            n242 = call "graph4.vi"("replay"="replay") -> ("y"=w391:dynamicdata, "x"=w392:dynamicdata, "size(s)"=→"size(s)":i32)  [unwired: 8 in]
            n243 = Bundle("Heading"=w397, "hgps"=w396) -> (→"Heading":cluster{"Heading":dbl, "hgps":dbl})  [unwired: 1 in]
            n244 = call "GRAPH2"("Y Input"=w391, "X Input"=w392) -> ("XY Graph"=→"XY Graph":cluster{"Y":dbl[], "Y":dbl[]}[])  [unwired: 3 in, 6 out]
          }
          frame #4 {
            n245 = global read "G_LCM.vi" "APP_GPS_DATA"() -> (w404:T12)
            n246 = Unbundle By Name(w404) -> ("Message"=w403:i64)
            n247 = Equal To 0?(x=w403) -> (x = 0?=w402:bool)
            n248 = case shown="1" w403 {
              tunnel: [_ TRUE _ _] -> _
              tunnel: [i32[] [0, 5, 0, 0] i32[] [1, 5, 0, 0] i32[] [0, 2, 0, 0] i32[] [0, 5, 3, 0]] -> w406
              frame 0, Default {
              }
              frame 1 {
              }
              frame 2 {
              }
              frame 3 {
              }
            }
            n249 = Select(t="", s=w402, f="미션중") -> (s? t:f=→"String":string)
            n250 = for {
              tunnel: w406 -> [w413] mode=indexing
              tunnel: [w412] -> w405 mode=indexing
              n251 = local read "sign 2"() -> (w414:picture[])
              n252 = Index Array(array=w414, index=w413) -> (element=w412:picture)
            }
            "P2V Sign" <- w405
          }
          frame #5 {
            n253 = global read "G_ALL.vi" "CARDATA"() -> (w421:T8)
            n254 = Unbundle By Name(w421) -> ("VS_des"=w424:dbl, "VS_can"=w431:dbl, "run"=w429:bool, "auto"=w430:bool, "Steer_input"=w416:dbl, "Steer_output"=w428:dbl)
            n255 = global read "G_ALL.vi" "Steering"() -> (w417:dbl)
            n256 = global read "G_ALL.vi" "VS_des"() -> (w420:dbl)
            n257 = Not(x=w429) -> (.not. x?=w433:bool)
            n258 = Add(x=w428, y=0.0) -> (x+y=w426:dbl)
            n259 = Negate(x=w416) -> (-x=w415:dbl)
            n260 = Select(t=w416, s=FALSE, f=w417) -> (s? t:f=w425:dbl)
            n261 = Select(t=w424, s=FALSE, f=w420) -> (s? t:f=w423:dbl)
            n262 = Bundle(w433, "auto"=w430) -> (w435:cluster{bool, "auto":bool})  [unwired: 1 in]
            n263 = Boolean To (0,1)(Boolean=w435) -> (0, 1=→"Waveform Chart 4":cluster{i16, "auto":i16})
            n264 = Bundle("VS_des"=w424, "VS_can"=w431, "VS_des"=w423) -> (→"Gauge":T4)  [unwired: 1 in]
            n265 = Bundle("VS_des"=w424, "VS_can"=w431, "VS_des"=w423) -> (→"Waveform Chart 2":T4)  [unwired: 1 in]
            n266 = Bundle(w415, w426, "Steering"=w425) -> (w437:cluster{dbl, dbl, "Steering":dbl})  [unwired: 1 in]
            n267 = Negate(x=w437) -> (-x=→"Meter" →"Waveform Chart 3":cluster{dbl, dbl, "Steering":dbl})
          }
          frame #6 {
            n268 = global read "G_ALL.vi" "CARDATA"() -> (w440:T8)
            n269 = global read "G_ALL.vi" "x origin"() -> (w439:dbl[])
            n270 = global read "G_ALL.vi" "y origin"() -> (w438:dbl[])
            n271 = call "Convert to Dynamic Data6"("Array"=w439) -> ("Dynamic Data Type"=w447:dynamicdata)  [unwired: 3 in]
            n272 = call "Convert to Dynamic Data7"("Array"=w438) -> ("Dynamic Data Type"=w446:dynamicdata)  [unwired: 3 in]
            n273 = Unbundle By Name(w440) -> ("x"=w444:dbl, "y"=w445:dbl)
            n274 = Merge Signals(w444, w447, w447) -> (w442:dynamicdata)
            n275 = Merge Signals(w445, w446, w446) -> (w441:dynamicdata)
            n276 = call "GRAPH"("Y Input"=w441, "X Input"=w442) -> ("XY Graph"=→"XY Graph 2":cluster{"Y":dbl[], "Y":dbl[]}[])  [unwired: 3 in, 6 out]
          }
        }
      }
      n277 = while {
        stop <- FALSE stop-if-true
        n278 = flat-sequence {
          frame #0 {
            # "Alert"
            n279 = Wait Until Next ms Multiple(millisecond multiple=u32 20 ("millisecond timer value")) -> ()  [unwired: 1 out]
          }
          frame #1 {
            n280 = global read "G_ALL.vi" "CARDATA"() -> (w348:T8)
            n281 = global read "G_ALL.vi" "beep"() -> (w349:T13)
            n282 = Unbundle By Name(w349) -> ("beep"=w346:bool, "frequency (Hz)"=w351:u32, "duration (msec)"=w350:u32)
            n283 = Unbundle By Name(w348) -> ("auto"=w347:bool)
            n284 = And(x=w347, y=w346) -> (x .and. y?=w345:bool)
            n285 = case shown="True" w345 {
              tunnel: w351 -> [_ w356]
              tunnel: w350 -> [_ w355]
              tunnel: w349 -> [_ w352]
              frame False {
              }
              frame True {
                w354 = FALSE ("use system alert? (T)")
                n286 = call <vilib>:"Beep.vi"("use system alert? (T)"=w354, "duration (msec)"=w355, "frequency (Hz)"=w356) -> ()  [unwired: 9 in]
                n287 = Bundle By Name(cluster=w352, "beep"=w354) -> (w353:T13)
                n288 = global write "G_ALL.vi" "beep"(w353) -> ()
              }
            }
          }
        }
      }
    }
  }
  n289 = flat-sequence {
    frame #0 {
      w450 = dbl[] [] ("x origin")
      w451 = 0.0 ("x")
      w452 = FALSE ("Make WPT")
      n290 = local write "mission auto"(TRUE ("mission auto")) -> ()
      n291 = local write "lane keep"(FALSE ("lane update")) -> ()
      n292 = local write "Global x shift"(w451) -> ()
      n293 = local write "obs shift"(w451) -> ()
      n294 = global write "G_ALL.vi" "x origin"(w450) -> ()
      n295 = global write "G_ALL.vi" "y origin"(w450) -> ()
      n296 = local write "Make WPT"(w452) -> ()
      n297 = local write "Load Path"(w452) -> ()
    }
    frame #1 {
      n298 = while {
        stop <- FALSE ("Loop 3") stop-if-true
        n299 = flat-sequence {
          frame #0 {
            n300 = Wait Until Next ms Multiple(millisecond multiple=u32 10 ("milliseconds to wait")) -> (millisecond timer value=w454:u32)
            n301 = feedback #5() -> (w456:u32)  [unwired: 1 in]
            n302 = feedback-in #5(w454) -> ()
            n303 = Subtract(x=w454, y=w456) -> (x-y=→"path":u32)
          }
          frame #1 {
            n304 = case shown="False" "Make WPT" {
              frame False {
                n305 = case shown="False" "Load Path" {
                  frame False {
                    n306 = flat-sequence {
                      frame #0 {
                        n307 = global read "G_ALL.vi" "x origin"() -> (w461:dbl[])
                        n308 = global read "G_SEN.vi" "M_lane_update"() -> (w462:bool)
                        n309 = Empty Array?(array=w461) -> (empty?=w460:bool)
                        n310 = case shown="True" w462 {
                          frame False {
                          }
                          frame True {
                            n311 = global read "G_SEN.vi" "M_lane_center"() -> (w524:dbl[])
                            n312 = Index Array(array=w524, index=10) -> (element=w530:dbl)
                            n313 = Multiply(x=w530, y=10.0) -> (x*y=w541:dbl)
                            n314 = Round Toward -Infinity(1:w541) -> (0:w527:dbl)
                            n315 = global read "G_SEN.vi" "y_mobileye"() -> (w521:dbl[])
                            n316 = Max & Min(x=100.0, y=w527) -> (max(x,y)=w544:dbl)  [unwired: 1 out]
                            n317 = Array Subset(array=w521, index=0, length=w544) -> (w503:dbl[])
                            n318 = Index Array(array=w524, index #1=7 ("index"), index #2=6 ("index"), index #3=9 ("index"), index #4=5 ("index")) -> (element #1=w525:dbl, element #2=w538:dbl, element #3=w536:dbl, element #4=w543:dbl)
                            n319 = Square(x=w503) -> (x^2=w532:dbl[])
                            n320 = Array Subset(array=w503, index=1) -> (w515:dbl[])  [unwired: 1 in]
                            n321 = Array Size(array=w515) -> (size(s)=w512:i32)
                            n322 = Compound Arithmetic op=MULTIPLY(w525, w503, w532) -> (w535:dbl[])
                            n323 = Compound Arithmetic op=MULTIPLY(w532, w538) -> (w534:dbl[])
                            n324 = Compound Arithmetic op=MULTIPLY(w503, w536) -> (w533:dbl[])
                            n325 = Compound Arithmetic op=ADD(w535, w534, w533, w543) -> (w502:dbl[])
                            n326 = Array Subset(array=w503, index=0, length=w512) -> (w514:dbl[])
                            n327 = Build Array(w502, w503) -> (w522:dbl[][])
                            n328 = Array Subset(array=w502, index=1) -> (w516:dbl[])  [unwired: 1 in]
                            n329 = Subtract(x=w515, y=w514) -> (x-y=w510:dbl[])
                            n330 = Array Size(array=w516) -> (size(s)=w519:i32)
                            n331 = Transpose 2D Array(2D array=w522) -> (transposed array=w523:dbl[][])
                            n332 = global write "G_ALL.vi" "map_track lane"(w523) -> ()
                            n333 = Array Subset(array=w502, index=0, length=w519) -> (w517:dbl[])
                            n334 = Subtract(x=w516, y=w517) -> (x-y=w509:dbl[])
                            n335 = Square(x=w510) -> (x^2=w508:dbl[])
                            n336 = Square(x=w509) -> (x^2=w507:dbl[])
                            n337 = Add(x=w508, y=w507) -> (x+y=w506:dbl[])
                            n338 = Square Root(x=w506) -> (sqrt(x)=w505:dbl[])
                            n339 = Build Array (concatenate)(w505, 0.0) -> (w501:dbl[])
                            n340 = global write "G_ALL.vi" "dist lane"(w501) -> ()
                          }
                        }
                        n341 = case shown="False" w460 {
                          frame False {
                            n342 = flat-sequence {
                              frame #0 {
                                w486 = 0.02 ("y")
                                # "Path Modify"
                                n343 = global read "G_ALL.vi" "CARDATA"() -> (w471:T8)
                                n344 = local read "obs shift"() -> (w488:dbl)
                                n345 = Unbundle By Name(w471) -> ("VS_can"=w470:dbl)
                                n346 = global read "G_ALL.vi" "OBS"() -> (w464:bool)
                                n347 = Absolute Value(x=w470) -> (abs(x)=w469:dbl)
                                n348 = Decrement(x=w486) -> (x-1=w484:dbl)
                                n349 = Select(t=w488, s=w464, f=0.0) -> (s? t:f=w478:dbl)
                                n350 = Multiply(x=w478, y=w486) -> (x*y=w485:dbl)
                                n351 = Less?(x=w469, y=2.0) -> (x < y?=w467:bool)
                                n352 = And(x="car detection", y=w467) -> (x .and. y?=w465:bool)
                                n353 = feedback #6() -> (w483:dbl)  [unwired: 1 in]
                                n354 = Multiply(x=w484, y=w483) -> (x*y=w482:dbl)
                                n355 = Subtract(x=w485, y=w482) -> (x-y=w481:dbl)
                                n356 = feedback-in #6(w481) -> ()
                                n357 = Multiply(x=0.1 ("y"), y="Global x shift") -> (x*y=w476:dbl)
                                n358 = Multiply(x="Globla y shift", y=0.1) -> (x*y=w474:dbl)
                                n359 = call "tracking4.vi"("y"=w474, "x"=w476, "reset path"="reset path", "d"="d", "car detection"=w465, "xt"=w481) -> ("mission"=w490:i32)  [unwired: 5 in]
                                n360 = Select(t=w490, s="mission auto", f="Mission") -> (s? t:f=w463:i32)
                                n361 = local write "Mission"(w463) -> ()
                                n362 = global write "G_ALL.vi" "mission num"(w463) -> ()
                              }
                              frame #1 {
                                w494 = 0.0 ("x")
                                n363 = global read "G_ALL.vi" "replay"() -> (w492:bool)
                                n364 = local write "car detection"(FALSE ("car detection")) -> ()
                                n365 = local write "Globla y shift"(w494) -> ()
                                n366 = local write "Global x shift"(w494) -> ()
                                n367 = case shown="False" w492 {
                                tunnel: [w497 _] -> w493
                                frame False {
                                n368 = local read "reset path"() -> (w496:bool)
                                n369 = case shown="False" w496 {
                                tunnel: [w499 _] -> w497
                                frame False {
                                n370 = call "obs_avoid.vi"("shifthold"="shifthold") -> ("obs shift"=w499:dbl)  [unwired: 10 in]
                                }
                                frame True {
                                n371 = local write "reset path"(FALSE ("reset path")) -> ()
                                }
                                }
                                }
                                frame True {
                                }
                                }
                                "obs shift" <- w493
                              }
                            }
                          }
                          frame True {
                          }
                        }
                      }
                      frame #1 {
                        n372 = global read "G_ALL.vi" "x origin"() -> (w549:dbl[])
                        n373 = Empty Array?(array=w549) -> (empty?=w548:bool)
                        n374 = Or(x="lane keep", y=w548) -> (x .or. y?=w550:bool)
                        n375 = call "path steer3.vi"("lane"=w550) -> ("curve vel limit"=w545:dbl, "handle"=w546:dbl)  [unwired: 9 in]
                        n376 = global write "G_ALL.vi" "Steering"(w546) -> ()
                        n377 = global write "G_ALL.vi" "curve vel limit"(w545) -> ()
                      }
                    }
                  }
                  frame True {
                    n378 = flat-sequence {
                      tunnel: [w566] -> w551
                      tunnel: w551 -> [w596]
                      frame #0 {
                        w553 = FALSE ("X Scale.Loose Fit")
                        w552 = u8 0 ("X Scale.Scale Fit")
                        n379 = call "initvar.vi"() -> ()  [unwired: 12 in]
                        n380 = property on="XY Graph" class="XYGraph (strict)"("XScale.ScaleFit"=w552, "YScale.ScaleFit"=w552, "XScale.LooseFit"=w553, "YScale.LooseFit"=w553) -> ()  [unwired: 2 in, 2 out]
                      }
                      frame #1 {
                        n381 = Bundle("Minimum"=-5.0, "Minimum"=37.3, "Minimum"=10.0, "Minimum"=1.0, "Minimum"=-20.0) -> (w558:T15)  [unwired: 1 in]
                        n382 = Bundle("Minimum"=-22.6, "Minimum"=22.6, "Minimum"=10.0, "Minimum"=1.0, "Minimum"=-20.0) -> (w565:T15)  [unwired: 1 in]
                        n383 = property on="XY Graph" class="XYGraph (strict)"("XScale.Range"=w565) -> ()  [unwired: 2 in, 2 out]
                        n384 = property on="XY Graph" class="XYGraph (strict)"("YScale.Range"=w558) -> ()  [unwired: 2 in, 2 out]
                      }
                      frame #2 {
                        n385 = global read "G_ALL.vi" "file path"() -> (w567:path)
                        n386 = Build Path(base path=w567, name or relative path="wpt") -> (appended path=w568:path)
                        n387 = call "Read From Measurement File2"("Filename"=w568, "Reset"=TRUE) -> ("error out"=w571:errorcluster, "Filename Out"=w566:path, "Signals"=w573:dynamicdata)  [unwired: 4 in, 3 out]
                        n388 = Unbundle By Name(w571) -> ("status"=w570:bool)
                        n389 = case shown="False" w570 {
                          tunnel: w573 -> [w574 _]
                          frame False {
                            n390 = call "Convert from Dynamic Data2"("Dynamic Data Type"=w574) -> ("Array"=w576:dbl[][])  [unwired: 3 in]
                            n391 = Empty Array?(array=w576) -> (empty?=w575:bool)
                            n392 = case shown="False" w575 {
                              tunnel: w576 -> [w583 _]
                              frame False {
                                n393 = Index Array(array=w583, index (row) #1=4 ("disabled index (col)"), index (row) #2=3 ("index (col)"), index (row) #3=7 ("index (row)")) -> (element #1=w582:dbl[], element #2=w581:dbl[], element #3=w577:dbl[])  [unwired: 3 in]
                                n394 = global write "G_ALL.vi" "x origin"(w582) -> ()
                                n395 = global write "G_ALL.vi" "y origin"(w581) -> ()
                                n396 = global write "G_ALL.vi" "mission"(w577) -> ()
                              }
                              frame True {
                                w584 = dbl[] [] ("x origin")
                                n397 = global write "G_ALL.vi" "x origin"(w584) -> ()
                                n398 = global write "G_ALL.vi" "y origin"(w584) -> ()
                              }
                            }
                          }
                          frame True {
                            w585 = dbl[] [] ("x origin")
                            n399 = global write "G_ALL.vi" "x origin"(w585) -> ()
                            n400 = global write "G_ALL.vi" "y origin"(w585) -> ()
                          }
                        }
                      }
                      frame #3 {
                        n401 = Strip Path(path=w596) -> (name=w592:string)  [unwired: 1 out]
                        n402 = local write "Load Path"(FALSE ("Load WPT")) -> ()
                        n403 = local write "reset path"(TRUE ("reset path")) -> ()
                        n404 = Match Pattern(string=w592, regular expression="_") -> (after substring=w594:string)  [unwired: 1 in, 3 out]
                        n405 = Match Pattern(string=w594, regular expression=".lvm") -> (before substring=w591:string)  [unwired: 1 in, 3 out]
                        n406 = Scan From String(input string=w591, default 1=T14."KAIST" ("map name")) -> (error out=w590:errorcluster, output 1=w588:T14)  [unwired: 3 in, 2 out]
                        n407 = case shown="Error" w590 {
                          tunnel: [w601 w602] -> w589
                          tunnel: w588 -> [w601 _]
                          frame No Error {
                          }
                          frame Error {
                            n408 = global read "G_ALL.vi" "GPSDATA"() -> (w603:T16)
                            n409 = Unbundle By Name(w603) -> ("map_idx"=w602:i32)
                          }
                        }
                        n410 = call "mapconf.vi"("map name"=w589) -> ("y"=w598:cluster{dbl, dbl, "y":dbl, "y":dbl, dbl}, "x"=w599:cluster{dbl, dbl, "y":dbl, "y":dbl, dbl}, "new picture"=w600:picture)  [unwired: 8 in]
                        n411 = property on="XY Graph 2" class="XYGraph (strict)"("PlotImages.Back"=w600) -> ()  [unwired: 2 in, 2 out]
                        n412 = property on="XY Graph 2" class="XYGraph (strict)"("XScale.Range"=w599, "YScale.Range"=w598) -> ()  [unwired: 2 in, 2 out]
                      }
                    }
                  }
                }
              }
              frame True {
                n413 = flat-sequence {
                  tunnel: [w607] -> w604
                  tunnel: w604 -> [w675]
                  frame #0 {
                    w605 = 0.0
                    n414 = global write "G_ALL.vi" "VS_des"(w605) -> ()
                    n415 = global write "G_ALL.vi" "Steering"(w605) -> ()
                  }
                  frame #1 {
                    n416 = local read "Make WPT"() -> (w606:bool)
                    n417 = Initialize Array(0.0 ("element"), 7 ("dimension size"), 1 ("dimension size")) -> (w608:dbl[][])
                    n418 = while {
                      shift-right: [w612] -> w607
                      shift-left: w608 -> [w614]
                      shift-right: [FALSE] -> _
                      shift-left: w606 -> [w615]
                      stop <- w617 stop-if-true
                      n419 = flat-sequence {
                        tunnel: [w629] -> w613
                        frame #0 {
                          n420 = global read "G_ALL.vi" "GPSDATA"() -> (w624:T16)
                          n421 = global read "G_ALL.vi" "CARDATA"() -> (w623:T8)
                          n422 = Unbundle By Name(w624) -> ("lat"=w628:dbl, "lon"=w627:dbl, "hgt"=w626:dbl, "map_idx"=w622:i32)
                          n423 = Unbundle By Name(w623) -> ("y"=w620:dbl, "x"=w619:dbl, "VS_can"=w621:dbl)
                          n424 = To Double Precision Float(number=w622) -> (double precision float=w625:dbl)
                          n425 = Build Array(w628, w627, w626, w620, w619, w626, w621, w625) -> (w629:dbl[])
                        }
                      }
                      n426 = local read "Make WPT"() -> (w618:bool)
                      n427 = Not(x=w618) -> (.not. x?=w617:bool)
                      n428 = case shown="False" w615 {
                        tunnel: w614 -> [w644 w661]
                        tunnel: w613 -> [w643 w659]
                        tunnel: [w642 w658] -> w612
                        frame False {
                          n429 = Array Size(array=w644) -> (size(s)=w652:i32[])
                          n430 = Index Array(array=w643, index #1=3 ("index"), index #2=4 ("index")) -> (element #1=w638:dbl, element #2=w636:dbl)
                          n431 = Index Array(array=w652, index=1) -> (element=w641:i32)
                          n432 = Decrement(x=w641) -> (x-1=w640:i32)
                          n433 = Index Array(array=w644, index (col)=w640) -> (element=w648:dbl[])  [unwired: 1 in]
                          n434 = Index Array(array=w648, index #1=3 ("index"), index #2=4 ("index")) -> (element #1=w639:dbl, element #2=w637:dbl)
                          n435 = Subtract(x=w639, y=w638) -> (x-y=w635:dbl)
                          n436 = Subtract(x=w637, y=w636) -> (x-y=w634:dbl)
                          n437 = Square(x=w635) -> (x^2=w633:dbl)
                          n438 = Square(x=w634) -> (x^2=w632:dbl)
                          n439 = Add(x=w633, y=w632) -> (x+y=w631:dbl)
                          n440 = Greater Or Equal?(x=w631, y=0.25) -> (x >= y?=w645:bool)
                          n441 = case shown="True" w645 {
                            tunnel: w644 -> [w653 w657]
                            tunnel: w641 -> [_ w654]
                            tunnel: w643 -> [_ w656]
                            tunnel: [w653 w655] -> w642
                            frame False {
                            }
                            frame True {
                              n442 = Insert Into Array(array=w657, index (col)=w654, new element=w656) -> (w655:dbl[][])  [unwired: 1 in]
                            }
                          }
                        }
                        frame True {
                          n443 = Replace Array Subset(array=w661, new element=w659, index (col)=0 ("disabled index (col)")) -> (w658:dbl[][])  [unwired: 1 in]
                        }
                      }
                    }
                  }
                  frame #2 {
                    n444 = call "Convert to Dynamic Data"("2D Array"=w675) -> ("Dynamic Data Type"=w676:dynamicdata)  [unwired: 3 in]
                    n445 = global read "G_ALL.vi" "GPSDATA"() -> (w665:T16)
                    n446 = Unbundle By Name(w665) -> ("map_idx"=w663:i32)
                    n447 = Get Date/Time In Seconds() -> (seconds since 1Jan1904=w673:timestamp)
                    n448 = Format Date/Time String(time format string (%c)="%2y%2m%2d%2H%2M", seconds (now)=w673) -> (date/time string=w671:string)  [unwired: 1 in]
                    n449 = Format Into String(w663) -> (resulting string=w662:string)  [unwired: 3 in, 1 out]
                    n450 = global read "G_ALL.vi" "file path"() -> (w664:path)
                    n451 = Build Path(base path=w664, name or relative path="wpt") -> (appended path=w668:path)
                    n452 = Concatenate Strings(w671, "_" ("string"), w662, ".lvm" ("string")) -> (w667:string)
                    n453 = Build Path(base path=w668, name or relative path=w667) -> (appended path=w666:path)
                    n454 = call "save wpt"("Signals"=w676, "Reset"=TRUE, "Filename"=w666) -> ()  [unwired: 14 in, 3 out]
                  }
                }
              }
            }
          }
        }
      }
    }
  }
